vi "WriteVersion.vi"(0 "session in":refnum<k35>, 5 "Data input":string, 7 "index":i32, 11 "error In":errorcluster) -> (4 "session out":refnum<k35>, 15 "error Out":errorcluster)   [LabVIEW 2023]
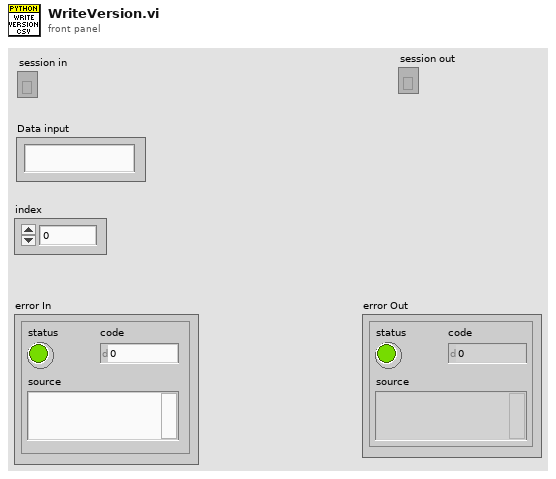
[diagram p1: front panel]
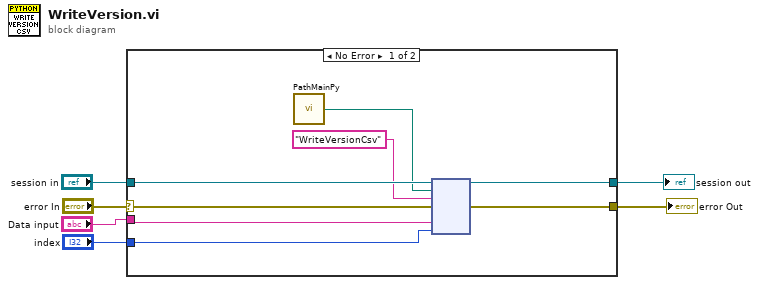
[diagram p0: block diagram]
diagram:
  n1 = case shown="No Error" "error In" {
    selector: "error In" -> [w13 w16]
    tunnel: [w11 w16] -> w1
    tunnel: "session in" -> [w12 w15]
    tunnel: [w10 w15] -> w2
    tunnel: "Data input" -> [w14 _]
    tunnel: "index" -> [w9 _]
    frame No Error {
      n2 = call "PathMainPy.vi"() -> ("path"=w7:path)  [unwired: 15 in]
      n3 = node(w12, w7, "WriteVersionCsv" ("Data input"), w13, w14, w9) -> (w10:refnum<k35>, w11:errorcluster)  [unwired: 4 in, 2 out]
    }
    frame Error {
    }
  }
  "session out" <- w2
  "error Out" <- w1
